vi "ShowWindowSystemMenu.vi"(8 "No Error":errorcluster, 9 "y":i32, 10 "x":i32, 11 "Window [SDL_Window *]":i64 format="%.0x") -> (0 "Error Out":errorcluster)   [LabVIEW 2024, in "SDL3.lvlib" / "Video.lvlib"]
doc: "<B>Summary</B>\nDisplay the system-level window menu.\n\n<B>Remarks</B>\nThis default window menu is provided by the system and on some platforms provides functionality for setting or changing privileged state on the window, such as moving it between workspaces or displays, or toggling the always-on-top property.\n\nOn platforms or desktops where this is unsupported, this function does nothing."
uses:
  Video.lvlib
  <vilib>/Utility/error.llb/Error Cluster From Error Code.vi
  Error/Error.lvlib
  Lib/SDL3-32.dll
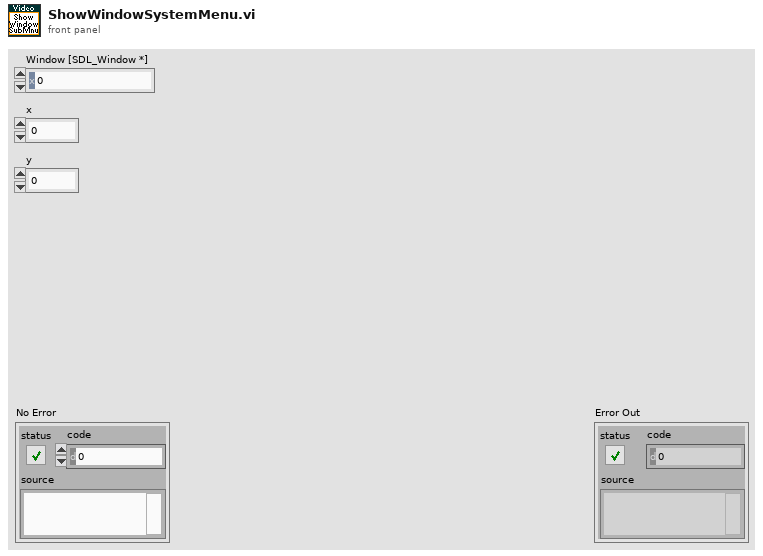
[diagram p1: front panel]
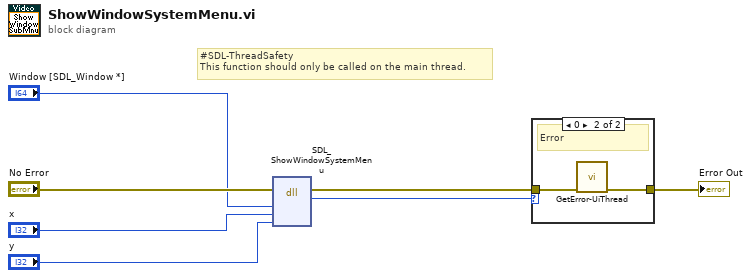
[diagram p0: block diagram]
diagram:
  # "#SDL-ThreadSafety\nThis function should only be called on the main thread."
  n1 = dll-call lib="C:/Users/Thomas/Documents/Projects/LV-SDL3/Lib/SDL3-*.*" fn="SDL_ShowWindowSystemMenu"(error in="No Error", "window"="Window [SDL_Window *]", "x"="x", "y"="y") -> (error out=w2:errorcluster, "return type"=w1:i32)  [unwired: 5 in, 1 out]
  n2 = case shown="0" w1 {
    tunnel: w2 -> [w8 w10]
    tunnel: [w8 w9] -> w6
    frame Default {
      # "Ok"
    }
    frame 0 {
      # "Error"
      n3 = call "GetError-UiThread.vi"("No Error"=w10) -> ("error out"=w9:errorcluster)  [unwired: 10 in]
    }
  }
  "Error Out" <- w6
